vi "Send Main to gRPC.vi"(8 "error in (no error)":errorcluster, 11 "CIFTemplatePlugin in":refnum<class "TemplatePlugin.lvclass">) -> (0 "error out":errorcluster, 3 "CIFTemplatePlugin out":refnum<class "TemplatePlugin.lvclass">)   [LabVIEW 2021, in "TemplatePlugin.lvclass"]
uses:
  TemplatePlugin.lvclass
  TemplatePlugin.lvclass/TemplatePlugin.ctl
  OOB/OOB_Tx/TemplateOOB_Tx.lvclass
  CIF-LVCore/src/CIFCore/Class/CIFCorePlugin.lvclass
  D:/dev/CIF-LVCore/src/CIFCore/Class/CIFCorePlugin.lvclass
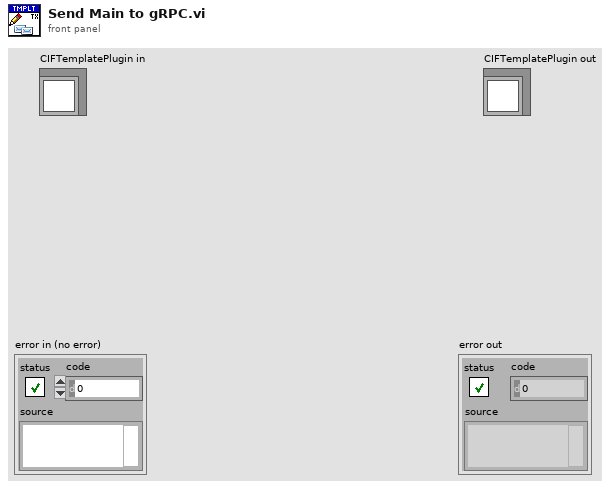
[diagram p1: front panel]
types:
  T1 = typedef "TemplatePlugin.lvclass/Main to gRPC Cyclic Data.ctl" = cluster{" Cyclic Data 1 ->gRPC":i32}
  T2 = typedef "TemplateOOB_Tx.lvclass/Main to gRPC Command Data.ctl" = cluster{"Cmd 1 Data -> gRPC":i32}
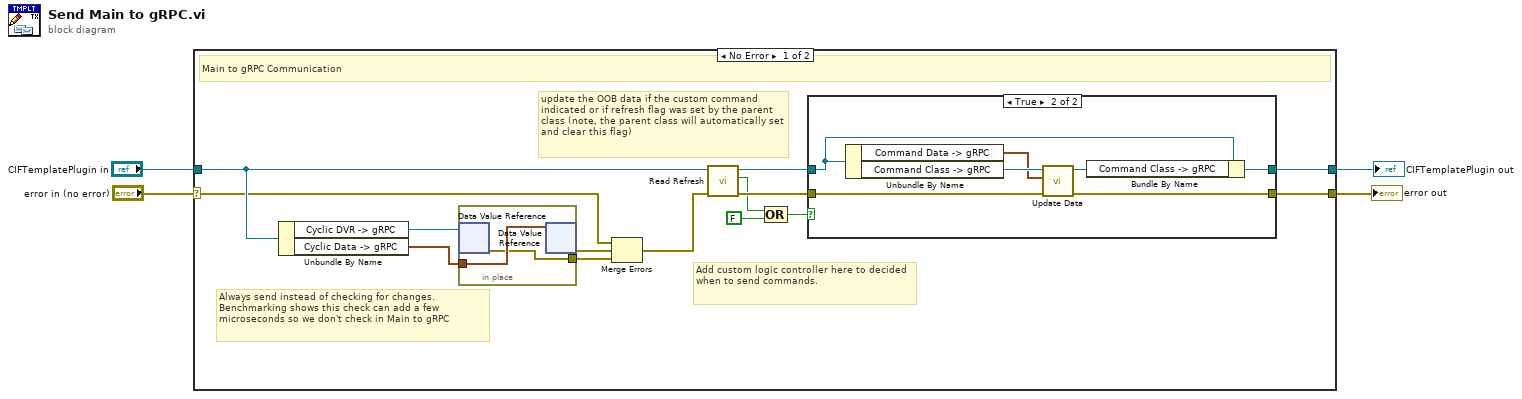
[diagram p0: block diagram]
diagram:
  n1 = case shown="No Error" "error in (no error)" {
    selector: "error in (no error)" -> [w8 w31]
    tunnel: [w17 w31] -> w3
    tunnel: [w18 w30] -> w1
    tunnel: "CIFTemplatePlugin in" -> [w9 w30]
    frame No Error {
      # "Always send instead of checking for changes.  Benchmarking shows this check can add a few microseconds so we don't check in Main to gRPC"
      # "Add custom logic controller here to decided when to send commands."
      # "update the OOB data if the custom command indicated or if refresh flag was set by the parent class (note, the parent class will automatically set and clear this flag)"
      # "Main to gRPC Communication"
      n2 = Unbundle By Name(w9) -> ("Cyclic DVR -> gRPC"=w13:refnum<data-value>, "Cyclic Data -> gRPC"=w10:T1)
      n3 = in-place {
        in-place-border: w10 -> [w20]
        in-place-border: [w19] -> w11
        n4 = in-place-dvr #1(w13) -> (w19:errorcluster)  [unwired: 1 out]
        n5 = in-place-dvr #1(w20) -> (w12:errorcluster)  [unwired: 1 out]
      }
      n6 = Merge Errors(w8, w12, w11) -> (w7:errorcluster)
      n7 = call "Read Refresh.vi"("error in (no error)"=w7, "CIFCorePlugin in"=w9) -> ("error out"=w15:errorcluster, "Refresh"=w14:bool, "CIFCorePlugin out"=w16:refnum<class "TemplatePlugin.lvclass">)  [unwired: 7 in]
      n8 = Compound Arithmetic op=OR(w14, FALSE ("value")) -> (w5:bool)
      n9 = case shown="True" w5 {
        tunnel: w15 -> [w21 w29]
        tunnel: w16 -> [w22 w28]
        tunnel: [w22 w27] -> w18
        tunnel: [w21 w26] -> w17
        frame False {
        }
        frame True {
          n10 = Unbundle By Name(w28) -> ("Command Data -> gRPC"=w23:T2, "Command Class -> gRPC"=w25:refnum<class "TemplateOOB_Tx.lvclass">)
          n11 = call "Update Data.vi"("error in"=w29, "Data"=w23, "CutomOOB_Tx in"=w25) -> ("error out"=w26:errorcluster, "CutomOOB_Tx out"=w24:refnum<class "TemplateOOB_Tx.lvclass">)  [unwired: 7 in]
          n12 = Bundle By Name(cluster=w28, "Command Class -> gRPC"=w24) -> (w27:refnum<class "TemplatePlugin.lvclass">)
        }
      }
    }
    frame Error {
    }
  }
  "error out" <- w3
  "CIFTemplatePlugin out" <- w1
